vi "calibrate_bemf_fisf.vi"(6 "timeout (25000ms)":i32=25000, 8 "error in (no error)":errorcluster, 10 "time wait ms":u32=3000, 11 "daemon reference in":refnum<k5>) -> (0 "error out":errorcluster, 1 "eol_cold_bemf_fisf":dbl, 2 "response":string, 3 "daemon reference out":refnum<k5>, 4 "eol_cold_bemf":dbl, 5 "command out":string="random")   [LabVIEW 2017]
doc: "<b>Command: </b>\"calibrate_bemf_fisf\"\n\n<b>Description: </b> This command instructure device start bemf fisf calibration.\n\n<b>Parameters: </b> time wait ms for bemf fisf calibration to complete\n____________________________________________\nDIPC 692 Daemon API 10.0.0.1\nSam Tee - Dyson Technology Ltd\nCopyright (c) 2024, Dyson Technology Ltd"
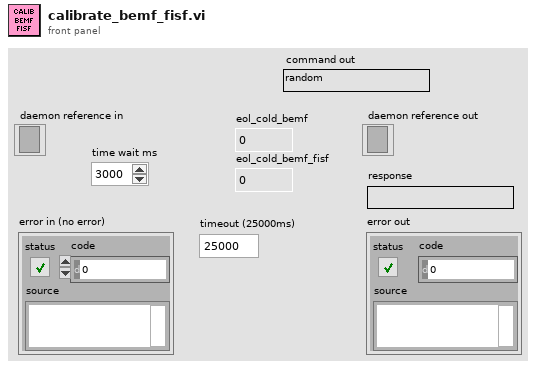
[diagram p1: front panel]
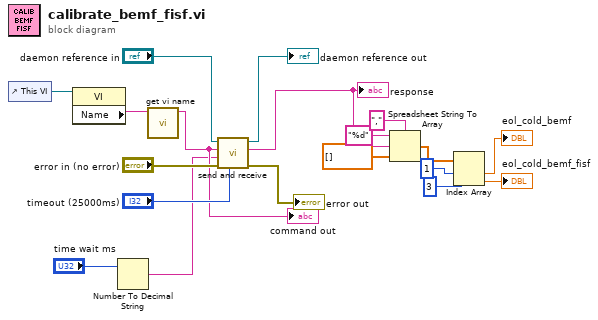
[diagram p0: block diagram]
diagram:
  n1 = control-ref of="This VI"() -> (w14:refnum<vi>)
  n2 = property class="VI"(reference=w14) -> ("Name"=w13:string)  [unwired: 1 in, 2 out]
  n3 = Number To Decimal String(number="time wait ms") -> (decimal integer string=w10:string)  [unwired: 1 in]
  n4 = call "get vi name.vi"("library.lvlib:name.vi"=w13) -> ("vi name"=w12:string)  [unwired: 10 in]
  "command out" <- w12
  n5 = call "send and receive.vi"("timeout (25000ms)"="timeout (25000ms)", "error in (no error)"="error in (no error)", "data"=w10, "command"=w12, "daemon reference in"="daemon reference in") -> ("error out"=→"error out":errorcluster, "response"=w8:string, "daemon reference out"=→"daemon reference out":refnum<k5>)  [unwired: 4 in]
  "response" <- w8
  n6 = Spreadsheet String To Array(delimiter (Tab)=",", format string="%d", spreadsheet string=w8, array type (2D Dbl)=dbl[] []) -> (array=w6:dbl[])
  n7 = Index Array(array=w6, index #1=1 ("index"), index #2=3 ("index")) -> (element #1=→"eol_cold_bemf":dbl, element #2=→"eol_cold_bemf_fisf":dbl)
